vi "Getmode.vi"(8 "error in (no error)":errorcluster, 11 "OneOfTemplate in":refnum<class "nixnet_grpc_CreateSessionRequest_mode_enum.lvclass">) -> (0 "error out":errorcluster, 2 "Get_Val":T1, 3 "OneOfTemplate out":refnum<class "nixnet_grpc_CreateSessionRequest_mode_enum.lvclass">)   [LabVIEW 2019, in "xnet-grpc_client.lvlib" / "nixnet_grpc_CreateSessionRequest_mode_enum.lvclass"]
uses:
  nixnet_grpc_CreateSessionRequest_mode_enum.lvclass
  nixnet_grpc_CreateSessionMode.ctl
  nixnet_grpc_CreateSessionRequest_mode_enum.lvclass/nixnet_grpc_CreateSessionRequest_mode_enum.ctl
  xnet-grpc_client.lvlib
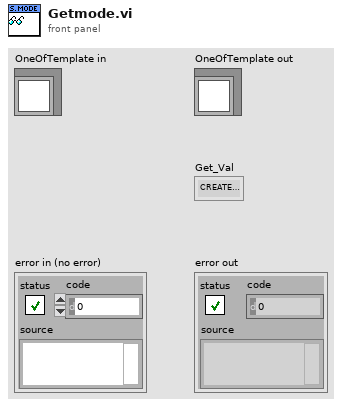
[diagram p1: front panel]
types:
  T1 = typedef "xnet-grpc_client.lvlib/nixnet_grpc_CreateSessionMode.ctl" = enum32{"CREATE_SESSION_MODE_SIGNAL_IN_SINGLE_POINT", "CREATE_SESSION_MODE_SIGNAL_IN_WAVEFORM", "CREATE_SESSION_MODE_SIGNAL_IN_XY", "CREATE_SESSION_MODE_SIGNAL_OUT_SINGLE_POINT", "CREATE_SESSION_MODE_SIGNAL_OUT_WAVEFORM", "CREATE_SESSION_MODE_SIGNAL_OUT_XY", "CREATE_SESSION_MODE_FRAME_IN_STREAM", "CREATE_SESSION_MODE_FRAME_IN_QUEUED", "CREATE_SESSION_MODE_FRAME_IN_SINGLE_POINT", "CREATE_SESSION_MODE_FRAME_OUT_STREAM", "CREATE_SESSION_MODE_FRAME_OUT_QUEUED", "CREATE_SESSION_MODE_FRAME_OUT_SINGLE_POINT", "CREATE_SESSION_MODE_SIGNAL_CONVERSION_SINGLE_POINT"}
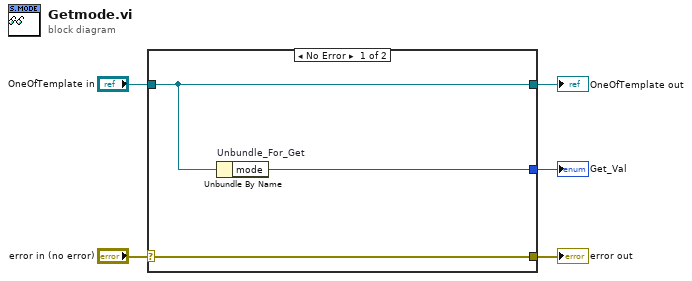
[diagram p0: block diagram]
diagram:
  n1 = case shown="No Error" "error in (no error)" {
    selector: "error in (no error)" -> [w8 w9]
    tunnel: [w8 w9] -> w4
    tunnel: [w7 w10] -> w2
    tunnel: "OneOfTemplate in" -> [w7 w10]
    tunnel: [w6 _] -> w1
    frame No Error {
      n2 = Unbundle By Name "Unbundle_For_Get"(w7) -> ("mode"=w6:T1)
    }
    frame Error {
    }
  }
  "error out" <- w4
  "OneOfTemplate out" <- w2
  "Get_Val" <- w1
